vi "Encode JSON Recursive.vi"(4 "error in (no error)":errorcluster, 6 "String In":string, 7 "JSON Tree":variant) -> (0 "error out":errorcluster, 2 "String Out":string)   [LabVIEW 2010, in "i3-json.lvlib"]
uses:
  i3-json.lvlib
  JSON Types/JSON Type.ctl
  Generation Error.ctl
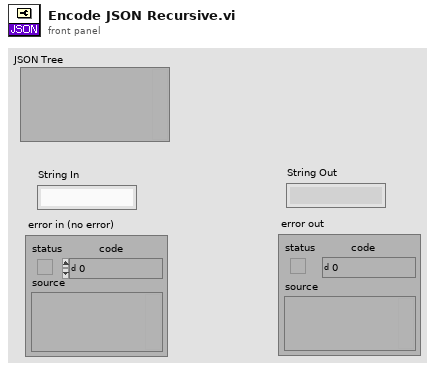
[diagram p1: front panel]
types:
  T1 = typedef "i3-json.lvlib/JSON Type.ctl" = enum8{"JSON Compatible", "JSON Array", "JSON Object", "JSON Null", "Double", "String", "Boolean", "Unknown"}
  T2 = typedef "i3-json.lvlib/Generation Error.ctl" = string
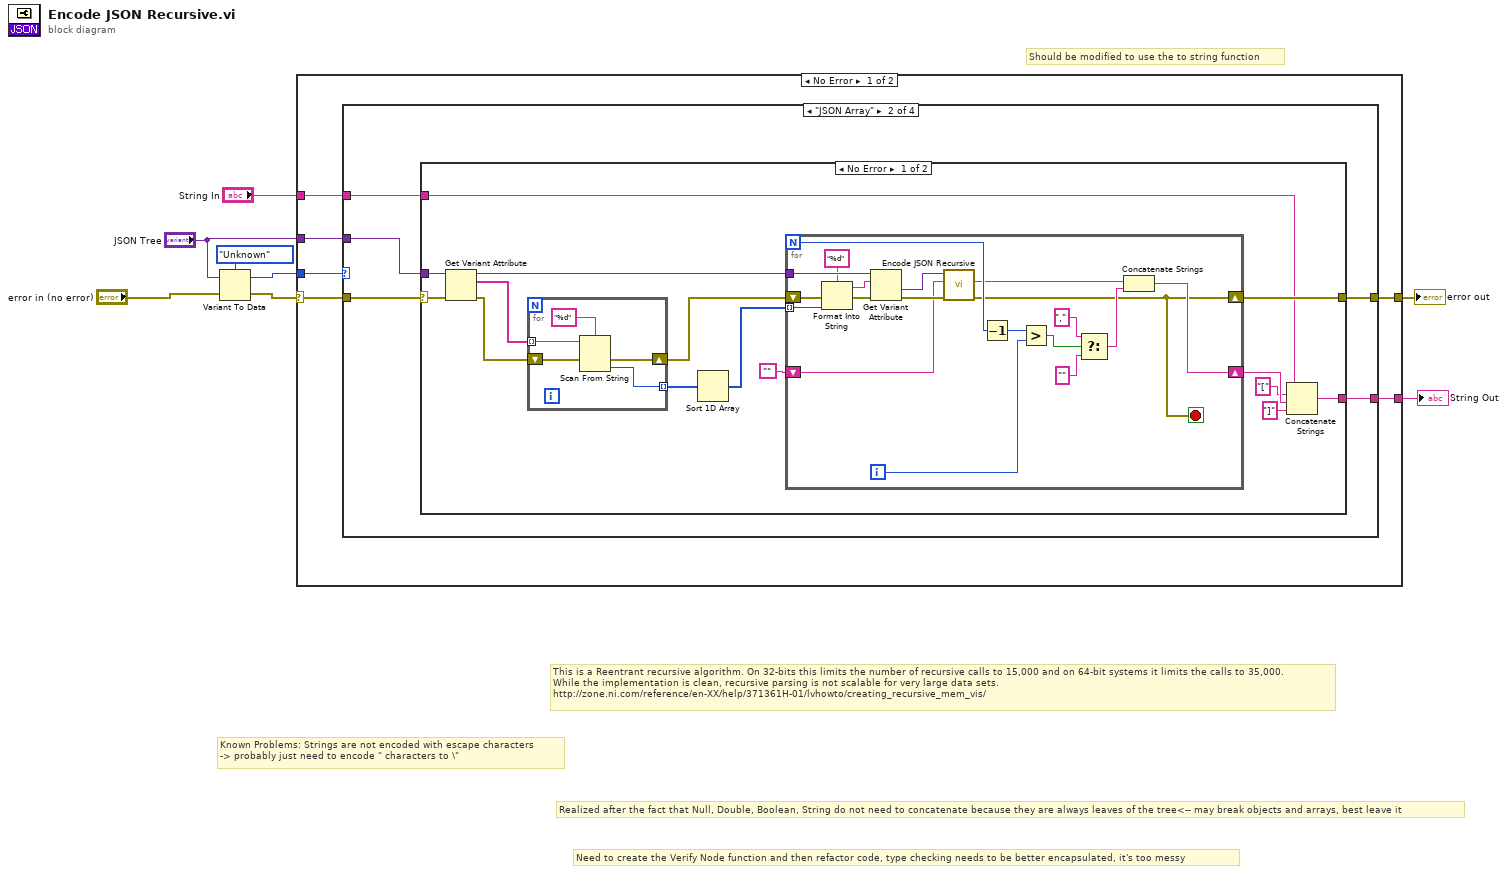
[diagram p0: block diagram]
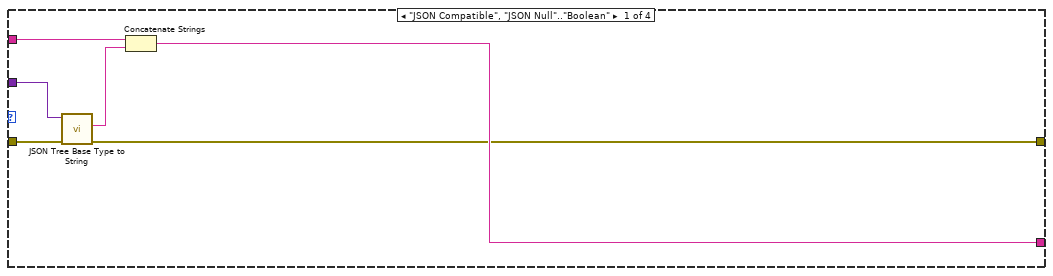
[diagram p2: hidden frame]
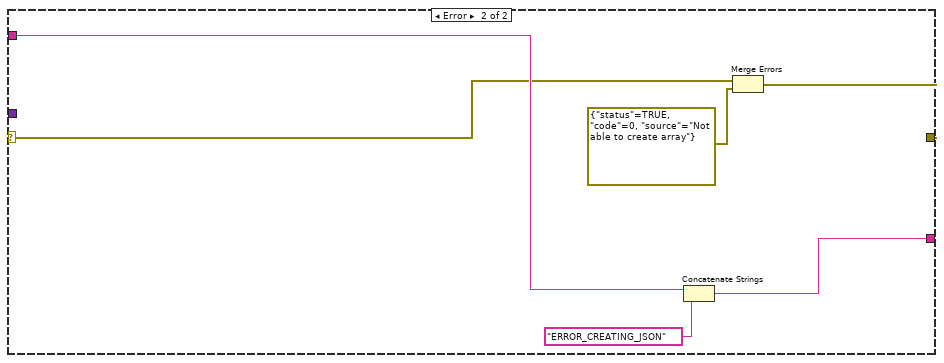
[diagram p3: hidden frame]
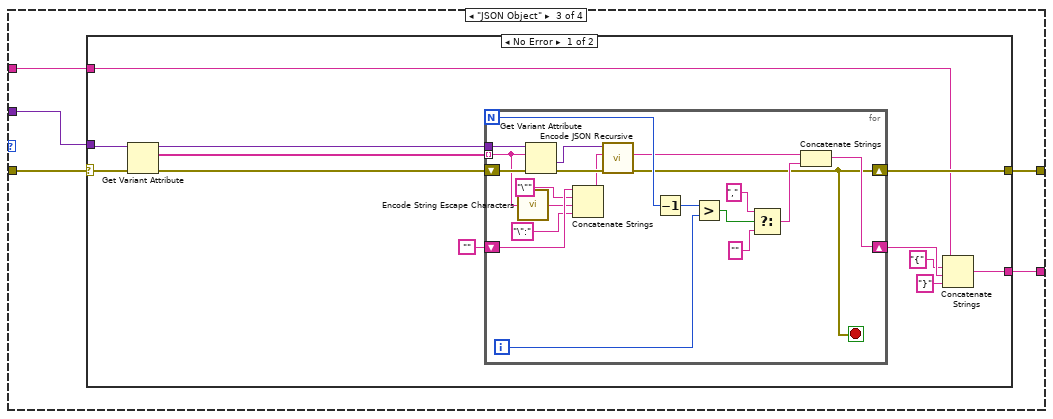
[diagram p4: hidden frame]
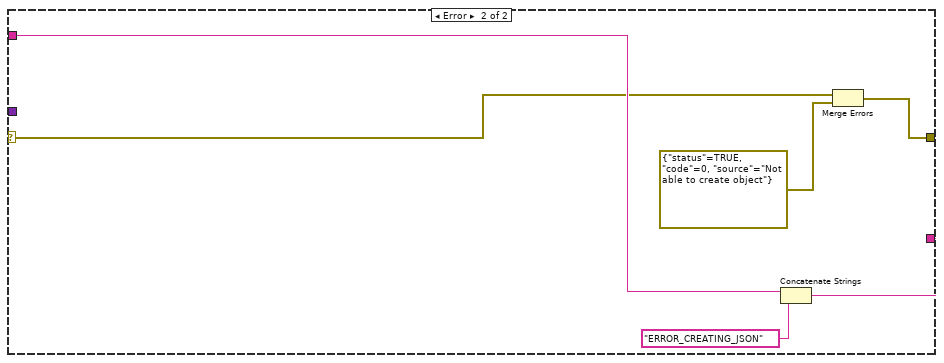
[diagram p5: hidden frame]
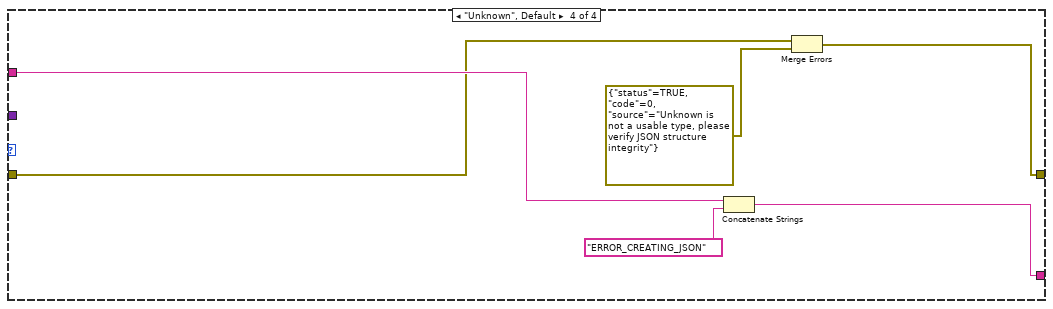
[diagram p6: hidden frame]
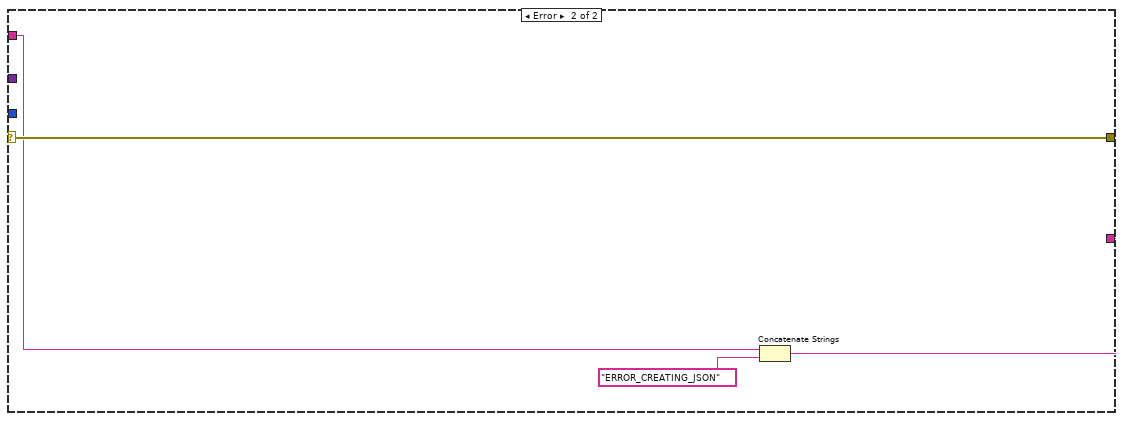
[diagram p7: hidden frame]
diagram:
  # "Should be modified to use the to string function"
  # "Need to create the Verify Node function and then refactor code, type checking needs to be better encapsulated, it's too messy"
  # "Realized after the fact that Null, Double, Boolean, String do not need to concatenate because they are always leaves of the tree<-- may break objects and arrays, best leave it"
  # "Known Problems: Strings are not encoded with escape characters\n-> probably just need to encode \" characters to \\\""
  # "This is a Reentrant recursive algorithm. On 32-bits this limits the number of recursive calls to 15,000 and on 64-bit systems it limits the calls to 35,000.\nWhile the implementation is clean, recursive parsing is not scalable for very large data sets.\nhttp://zone.ni.com/reference/en-XX/help/371361H-01/lvhowto/creating_recursive_mem_vis/"
  n1 = Variant To Data(error in="error in (no error)", Variant="JSON Tree", type=JSON_Type."Unknown" ("JSON Type")) -> (error out=w6:errorcluster, data=w5:T1)
  n2 = case shown="No Error" w6 {
    selector: w6 -> [w12 w123]
    tunnel: w5 -> [w14 _]
    tunnel: "JSON Tree" -> [w13 _]
    tunnel: "String In" -> [w11 w122]
    tunnel: [w10 w121] -> w3
    tunnel: [w9 w123] -> w2
    frame No Error {
      n3 = case shown="\"JSON Array\"" w14 {
        tunnel: w13 -> [w15 w22 w75 _]
        tunnel: w12 -> [w16 w24 w71 w114]
        tunnel: w11 -> [w20 w23 w74 w118]
        tunnel: [w18 w21 w73 w117] -> w10
        tunnel: [w17 w25 w72 w116] -> w9
        frame "JSON Compatible", "JSON Null".."Boolean" {
          n4 = call "JSON Tree Base Type to String.vi"("error in (no error)"=w16, "JSON Tree Base Type"=w15) -> ("error out"=w17:errorcluster, "JSON Tree Base Type String"=w19:string)  [unwired: 8 in]
          n5 = Concatenate Strings(w20, w19) -> (w18:string)
        }
        frame "JSON Array" {
          n6 = case shown="No Error" w24 {
            selector: w24 -> [w39 w65]
            tunnel: [w36 w70] -> w25
            tunnel: w23 -> [w31 w69]
            tunnel: [w33 w67] -> w21
            tunnel: w22 -> [w40 _]
            frame No Error {
              n7 = Get Variant Attribute(Variant=w40, error in=w39) -> (duplicate Variant=w38:variant, names=w29:string[], error out=w26:errorcluster)  [unwired: 2 in, 1 out]
              n8 = for {
                tunnel: w29 -> [w45] mode=indexing
                shift-right: [w43] -> w27
                shift-left: w26 -> [w44]
                tunnel: [w42] -> w28 mode=indexing
                n9 = Scan From String(format string="%d", input string=w45, error in=w44) -> (error out=w43:errorcluster, output 1=w42:i32)  [unwired: 2 in, 2 out]
              }
              n10 = Sort 1D Array(array=w28) -> (sorted array=w37:i32[])
              n11 = for {
                N -> [w61]
                tunnel: w38 -> [w64]
                tunnel: w37 -> [w48] mode=indexing
                shift-right: [w51] -> w36
                shift-left: w27 -> [w49]
                shift-right: [w53] -> w35
                shift-left: "" -> [w52]
                i -> [w55]
                stop <- w51 stop-if-true
                n12 = Format Into String(format string="%d", error in=w49, w48) -> (resulting string=w46:string, error out=w50:errorcluster)  [unwired: 1 in]
                n13 = Get Variant Attribute(Variant=w64, name=w46, error in=w50) -> (value=w62:variant, error out=w63:errorcluster)  [unwired: 1 in, 2 out]
                n14 = call "Encode JSON Recursive.vi"("error in (no error)"=w63, "String In"=w52, "JSON Tree"=w62) -> ("error out"=w51:errorcluster, "String Out"=w57:string)  [unwired: 3 in]
                n15 = Decrement(x=w61) -> (x-1=w54:i32)
                n16 = Greater?(x=w54, y=w55) -> (0:w60:bool)
                n17 = Select(t=",", s=w60, f="") -> (s? t:f=w56:string)
                n18 = Concatenate Strings(w57, w56) -> (w53:string)
              }
              n19 = Concatenate Strings(w31, "[" ("string"), w35, "]" ("string")) -> (w33:string)
            }
            frame Error {
              n20 = Concatenate Strings(w69, T2 "ERROR_CREATING_JSON" ("Generating Error")) -> (w67:string)
              n21 = Merge Errors(w65, errorcluster {"status"=TRUE, "code"=0, "source"="Not able to create array"} ("error in")) -> (w70:errorcluster)
            }
          }
        }
        frame "JSON Object" {
          n22 = case shown="No Error" w71 {
            selector: w71 -> [w86 w108]
            tunnel: [w83 w113] -> w72
            tunnel: w74 -> [w78 w112]
            tunnel: [w80 w110] -> w73
            tunnel: w75 -> [w87 _]
            frame No Error {
              n23 = Get Variant Attribute(Variant=w87, error in=w86) -> (duplicate Variant=w85:variant, names=w77:string[], error out=w84:errorcluster)  [unwired: 2 in, 1 out]
              n24 = for {
                N -> [w103]
                tunnel: w85 -> [w107]
                shift-right: [w90] -> w83
                shift-left: w84 -> [w106]
                shift-right: [w95] -> w82
                shift-left: "" -> [w94]
                tunnel: w77 -> [w88] mode=indexing
                i -> [w97]
                stop <- w90 stop-if-true
                n25 = call "Encode String Escape Characters.vi"("unescaped string in"=w88) -> ("escaped string out"=w89:string)
                n26 = Get Variant Attribute(Variant=w107, name=w88, error in=w106) -> (value=w104:variant, error out=w105:errorcluster)  [unwired: 1 in, 2 out]
                n27 = Concatenate Strings(w94, "\"" ("string"), w89, "\":" ("string")) -> (w91:string)
                n28 = call "Encode JSON Recursive.vi"("error in (no error)"=w105, "String In"=w91, "JSON Tree"=w104) -> ("error out"=w90:errorcluster, "String Out"=w99:string)  [unwired: 3 in]
                n29 = Decrement(x=w103) -> (x-1=w96:i32)
                n30 = Greater?(x=w96, y=w97) -> (0:w102:bool)
                n31 = Select(t=",", s=w102, f="") -> (s? t:f=w98:string)
                n32 = Concatenate Strings(w99, w98) -> (w95:string)
              }
              n33 = Concatenate Strings(w78, "{" ("string"), w82, "}" ("string")) -> (w80:string)
            }
            frame Error {
              n34 = Concatenate Strings(w112, T2 "ERROR_CREATING_JSON" ("Generating Error")) -> (w110:string)
              n35 = Merge Errors(w108, errorcluster {"status"=TRUE, "code"=0, "source"="Not able to create object"} ("error in")) -> (w113:errorcluster)
            }
          }
        }
        frame "Unknown", Default {
          n36 = Concatenate Strings(w118, T2 "ERROR_CREATING_JSON" ("Generating Error")) -> (w117:string)
          n37 = Merge Errors(w114, errorcluster {"status"=TRUE, "code"=0, "source"="Unknown is not a usable type, please verify JSON structure integrity"} ("error in")) -> (w116:errorcluster)
        }
      }
    }
    frame Error {
      n38 = Concatenate Strings(w122, T2 "ERROR_CREATING_JSON" ("string")) -> (w121:string)
    }
  }
  "String Out" <- w3
  "error out" <- w2
